vi "ArmSetLEDemand.vi"(9 "SetExtendPositonDemand(in)":dbl, 10 "SetLIftPostionDemand(d)":dbl) -> ()   [LabVIEW 2020]
doc: "Setters for Arm\nInputs:\n--SetRotatePositionDemand(d)--\n--SetLiftPostionDemand(d)--\n--SetExtendPostionDemand(in)--"
uses:
  ArmGlobal.vi
  <vilib>/Rock Robotics/WPI/ThirdParty/JAS_Junk/TrajLib/Trajectory_Library.lvlib
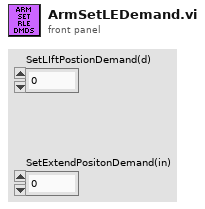
[diagram p1: front panel]
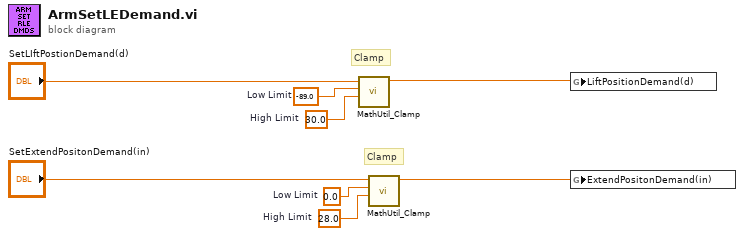
[diagram p0: block diagram]
diagram:
  w1 = -89.0  # Low Limit
  w4 = 30.0  # High Limit
  w8 = 28.0  # High Limit
  w7 = 0.0  # Low Limit
  # "Clamp"
  # "Clamp"
  n1 = call <vilib>:"MathUtil_Clamp.vi"("High Limit"=w4, "Low Limit"=w1, "Value"="SetLIftPostionDemand(d)") -> ("Result"=w2:dbl)  [unwired: 8 in]
  n2 = call <vilib>:"MathUtil_Clamp.vi"("High Limit"=w8, "Low Limit"=w7, "Value"="SetExtendPositonDemand(in)") -> ("Result"=w5:dbl)  [unwired: 8 in]
  n3 = global write "ArmGlobal.vi" "LiftPositionDemand(d)"(w2) -> ()
  n4 = global write "ArmGlobal.vi" "ExtendPositonDemand(in)"(w5) -> ()
